vi "Get Parallel Tests Enabled.vi"(8 "error in (no error)":errorcluster, 11 "Configuration Manager In":refnum<class "Configuration Manager.lvclass">) -> (0 "error out":errorcluster, 2 "Parallel tetss enabled?":bool, 3 "Configuration Manager Out":refnum<class "Configuration Manager.lvclass">)   [LabVIEW 2020, in "Configuration Manager.lvclass"]
uses:
  Configuration Manager.lvclass
  Configuration Manager.lvclass/Configuration Manager.ctl
  <vilib>/Utility/config.llb/Read Key (Boolean).vi
  <vilib>/Utility/config.llb/Write Key (Boolean).vi
  <vilib>/Utility/config.llb/NI_LVConfig.lvlib
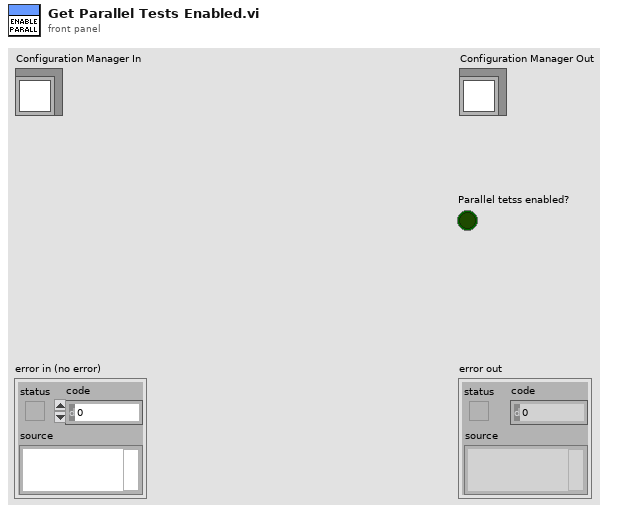
[diagram p1: front panel]
types:
  T1 = typedef "NI_LVConfig.lvlib/Config Data RefNum.ctl" = refnum<k1>
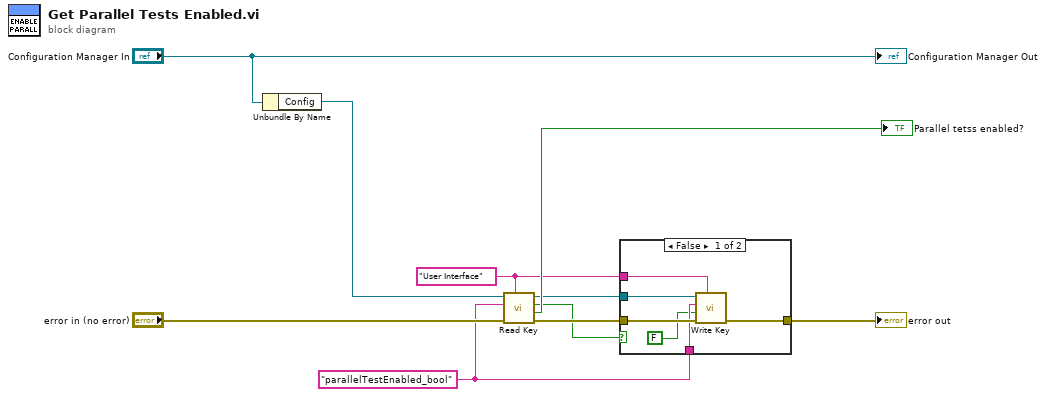
[diagram p0: block diagram]
diagram:
  w2 = "parallelTestEnabled_bool" ("key")
  w1 = "User Interface" ("section")
  n1 = Unbundle By Name("Configuration Manager In") -> ("Config"=w8:T1)
  n2 = call-poly <vilib>:"Read Key.vi"("section"=w1, "error in (no error)"="error in (no error)", "key"=w2, "refnum"=w8) -> ("error out"=w9:errorcluster, "value"=→"Parallel tetss enabled?":bool, "found?"=w4:bool, "refnum out"=w3:T1)  [unwired: 4 in]
  n3 = case shown="False" w4 {
    tunnel: w9 -> [w16 w17]
    tunnel: [w15 w17] -> w5
    tunnel: w3 -> [w14 _]
    tunnel: w2 -> [w13 _]
    tunnel: w1 -> [w11 _]
    frame False {
      n4 = call-poly <vilib>:"Write Key.vi"("section"=w11, "error in (no error)"=w16, "value"=FALSE, "key"=w13, "refnum"=w14) -> ("error out"=w15:errorcluster)  [unwired: 4 in, 2 out]
    }
    frame True {
    }
  }
  "error out" <- w5
  "Configuration Manager Out" <- "Configuration Manager In"
